vi "myRIO_BRig_RT_dataTrial_LeftRight.vi"() -> (2 "output_LeftRight":i32)   [LabVIEW 2014]
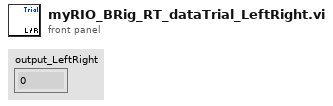
[diagram p1: front panel]
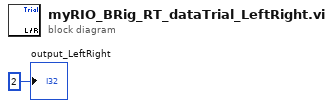
[diagram p0: block diagram]
diagram:
  "output_LeftRight" <- 2 ("output_iBlock")
